vi "Try X Tovey Receive.vi"(8 "error in (no error)":errorcluster, 11 "Model in":refnum<class "Model.lvclass">) -> (0 "error out":errorcluster, 2 "Data Present":bool, 3 "Model out":refnum<class "Model.lvclass">)   [LabVIEW 2016]
uses:
  TEI-9150/Tovey 9150.lvclass
  Model.lvclass
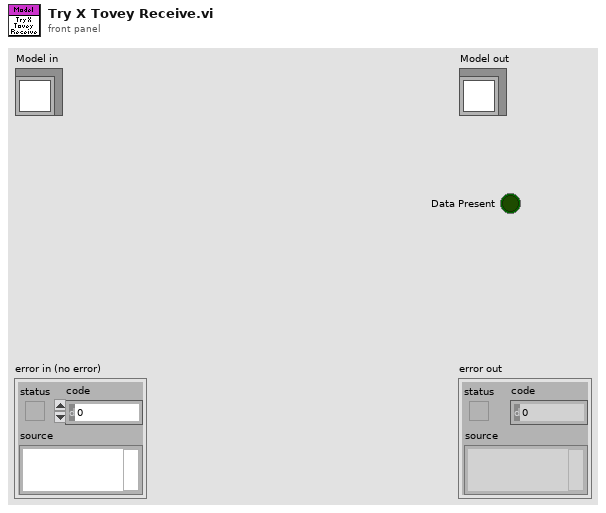
[diagram p1: front panel]
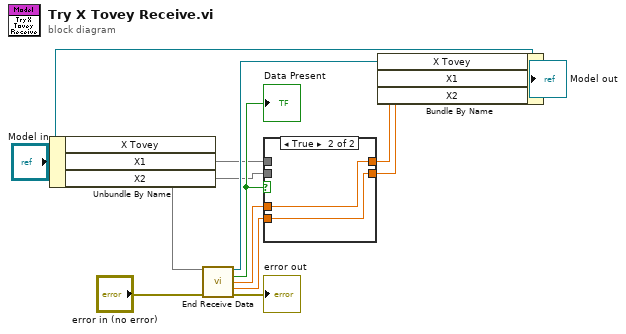
[diagram p0: block diagram]
diagram:
  n1 = Unbundle By Name("Model in") -> ("X Tovey"=w11, "X1"=w8, "X2"=w6)
  n2 = call "End Receive Data.vi"("Tovey9150 in"=w11, "error in (no error)"="error in (no error)") -> ("Tovey9150 out"=w10:refnum<class "Tovey 9150.lvclass">, "Data Present"=w9:bool, "A"=w4:dbl, "B"=w3:dbl, "error out"=→"error out":errorcluster)  [unwired: 9 in]
  "Data Present" <- w9
  n3 = case shown="True" w9 {
    tunnel: w8 -> [w15 _]
    tunnel: [w15 w17] -> w7
    tunnel: w6 -> [w14 _]
    tunnel: [w14 w16] -> w5
    tunnel: w4 -> [_ w17]
    tunnel: w3 -> [_ w16]
    frame False {
    }
    frame True {
    }
  }
  n4 = Bundle By Name(cluster="Model in", "X Tovey"=w10, "X1"=w7, "X2"=w5) -> (→"Model out":cluster{})
